vi "filter_mass_data.vi"(11 "Data In":string) -> (3 "Data Out":string)   [LabVIEW 2018, in "Labview Python.lvlib"]
uses:
  Labview Python.lvlib
  Post Analysis/Post-Analysis/Post Experiment Mass Analysis/Controls/Scan Information.ctl
  Mass Analysis/Preprocessing/Data.ctl
  Mass Analysis/Mass Analysis.lvlib
  Post Analysis/Post Analysis.lvlib
panel:
  out "JSON string":string
  in  "output cluster":T1
  in  "Cluster":T2={"High Frequency (Hz)"=[], "Low Frequency (Hz)"=[], "Peak Width"=[], "Peak Amplitude"=[], "UV Lamp"=[], "Time (s)"=[], "Fit Position (Hz)"=[], "Mass To Charge (kg/e)"=[], "Charge (e)"=[], "Window Size"=10.0, "Max Sweep Range"=500.0} {"Max Sweep Range" format="%#_13g"}
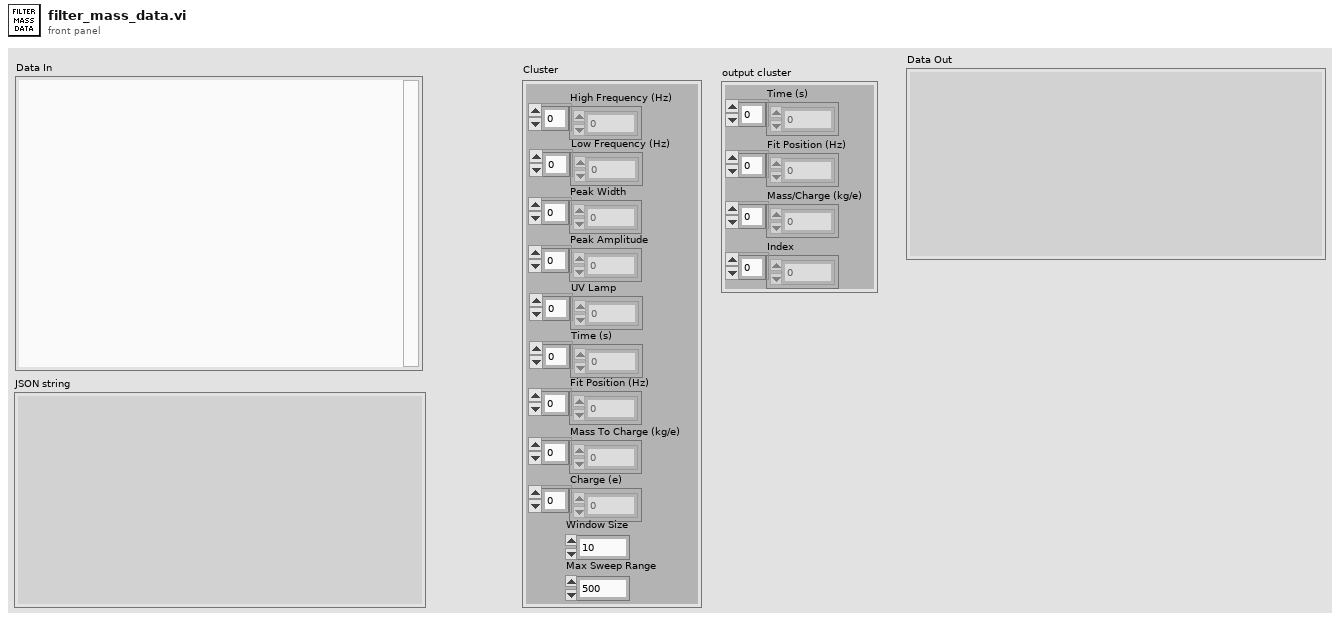
[diagram p1: front panel]
types:
  T1 = cluster{"Time (s)":dbl[], "Fit Position (Hz)":dbl[], "Mass/Charge (kg/e)":dbl[], "Index":i32[]}
  T2 = cluster{"High Frequency (Hz)":dbl[], "Low Frequency (Hz)":dbl[], "Peak Width":dbl[], "Peak Amplitude":dbl[], "UV Lamp":dbl[], "Time (s)":dbl[], "Fit Position (Hz)":dbl[], "Mass To Charge (kg/e)":dbl[], "Charge (e)":dbl[], "Window Size":dbl, "Max Sweep Range":dbl}
  T3 = typedef "Mass Analysis.lvlib/Data.ctl" = cluster{"Time (s)":dbl[], "Fit Position (Hz)":dbl[], "Mass To Charge (kg/e)":dbl[], "Charge (e)":dbl[]}
  T4 = typedef "Post Analysis.lvlib/Scan Information.ctl" = cluster{"High Frequency (Hz)":dbl[], "Peak Width":dbl[], "Peak Amplitude":dbl[], "Low Frequency (Hz)":dbl[], "UV Lamp":bool[]}
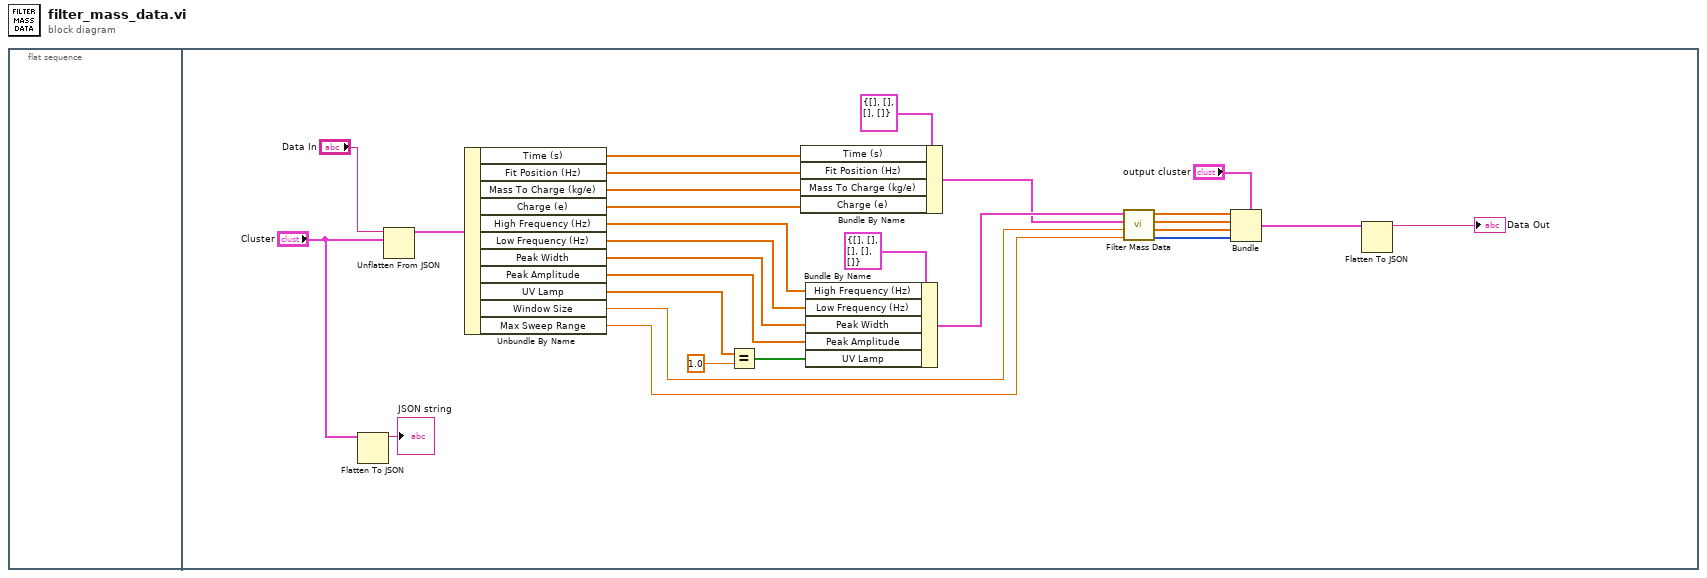
[diagram p0: block diagram]
diagram:
  n1 = flat-sequence {
    frame #0 {
    }
    frame #1 {
      n2 = Flatten To JSON(anything="Cluster") -> (JSON string=→"JSON string":string)  [unwired: 2 in, 1 out]
      n3 = Unflatten From JSON(JSON string="Data In", type and defaults="Cluster") -> (value=w26:T2)  [unwired: 5 in, 1 out]
      n4 = Unbundle By Name(w26) -> ("Time (s)"=w24:dbl[], "Fit Position (Hz)"=w23:dbl[], "Mass To Charge (kg/e)"=w22:dbl[], "Charge (e)"=w21:dbl[], "High Frequency (Hz)"=w20:dbl[], "Low Frequency (Hz)"=w19:dbl[], "Peak Width"=w18:dbl[], "Peak Amplitude"=w17:dbl[], "UV Lamp"=w14:dbl[], "Window Size"=w4:dbl, "Max Sweep Range"=w3:dbl)
      n5 = Equal?(x=w14, y=1.0) -> (x = y?=w12:bool[])
      n6 = Bundle By Name(cluster=T3 {"Time (s)"=[], "Fit Position (Hz)"=[], "Mass To Charge (kg/e)"=[], "Charge (e)"=[]} ("Data"), "Time (s)"=w24, "Fit Position (Hz)"=w23, "Mass To Charge (kg/e)"=w22, "Charge (e)"=w21) -> (w15:T3)
      n7 = Bundle By Name(cluster=T4 {"High Frequency (Hz)"=[], "Peak Width"=[], "Peak Amplitude"=[], "Low Frequency (Hz)"=[], "UV Lamp"=[]} ("Scan Information"), "High Frequency (Hz)"=w20, "Low Frequency (Hz)"=w19, "Peak Width"=w18, "Peak Amplitude"=w17, "UV Lamp"=w12) -> (w16:T4)
      n8 = call "Filter Mass Data.vi"("Max Sweep Range"=w3, "Window Size"=w4, "Data"=w15, "Scan Information"=w16) -> ("Index Out"=w7:i32[], "M/Q (kg/s) Out"=w8:dbl[], "Fit Position (Hz) Out"=w9:dbl[], "Time (s) Out"=w10:dbl[])  [unwired: 4 in]
      n9 = Bundle(cluster="output cluster", "Time (s)"=w10, "Fit Position (Hz)"=w9, "Mass/Charge (kg/e)"=w8, "Index"=w7) -> (w6:T1)
      n10 = Flatten To JSON(anything=w6) -> (JSON string=→"Data Out":string)  [unwired: 2 in, 1 out]
    }
  }
